vi "Simple VISA Terminal.vi"() -> ()   [LabVIEW 2025]
doc: "Simple string based state machine with internal error handling.\n\n--------------------\n<Author>\n<Company>"
uses:
  <vilib>/Utility/error.llb/Error Cluster From Error Code.vi
  <vilib>/Instr/_visa.llb/VISA Configure Serial Port (Instr).vi
  <vilib>/ErrorRing/Error Ring.xnode
panel:
  in  "Query":bool
  in  "Read":bool
  in  "Write":bool
  in  "VISA resource name":refnum<visa-resource-name>
  in  "Stop":bool
  in  "Start":bool
  in  "Command":string
  out "Error Out":errorcluster
  in  "Error In":errorcluster
  out "Reply":string
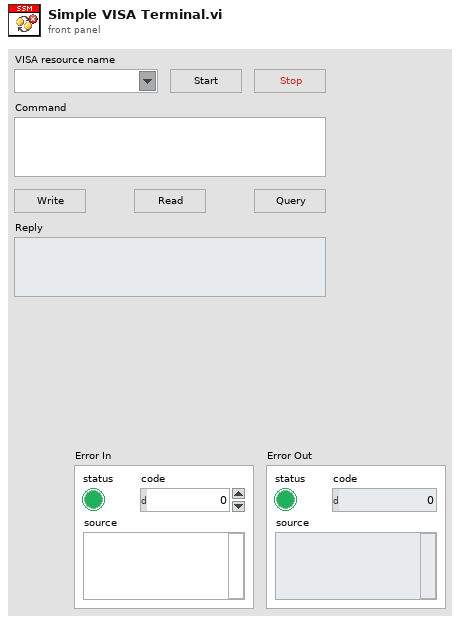
[diagram p1: front panel]
types:
  T1 = cluster{"VISA Reference":refnum<visa-resource-name>, "Reply":string, "Command":string, "Query?":bool}
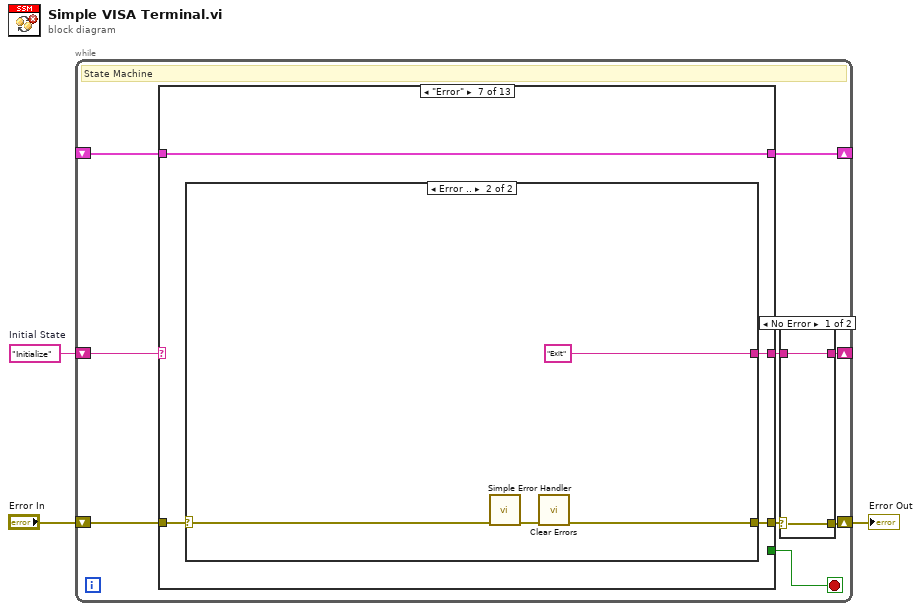
[diagram p0: block diagram]
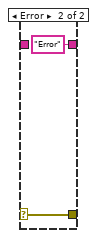
[diagram p2: hidden frame]
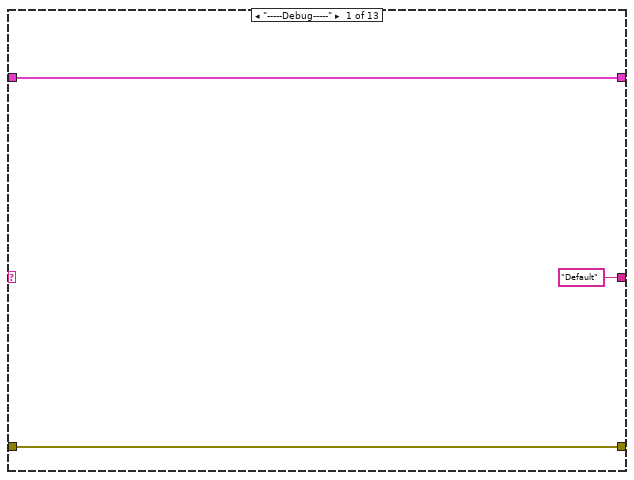
[diagram p3: hidden frame]
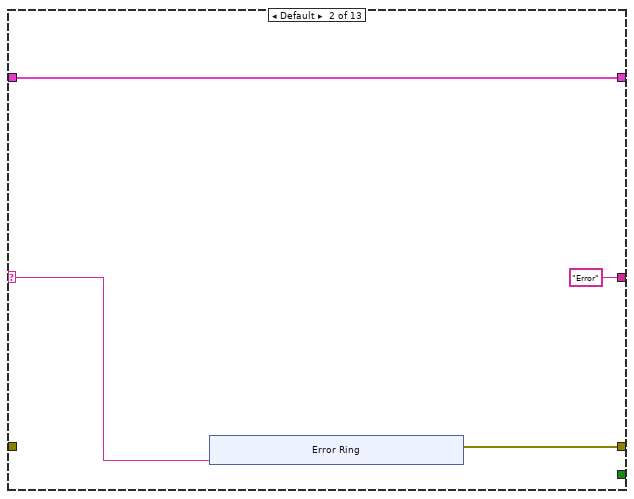
[diagram p4: hidden frame]
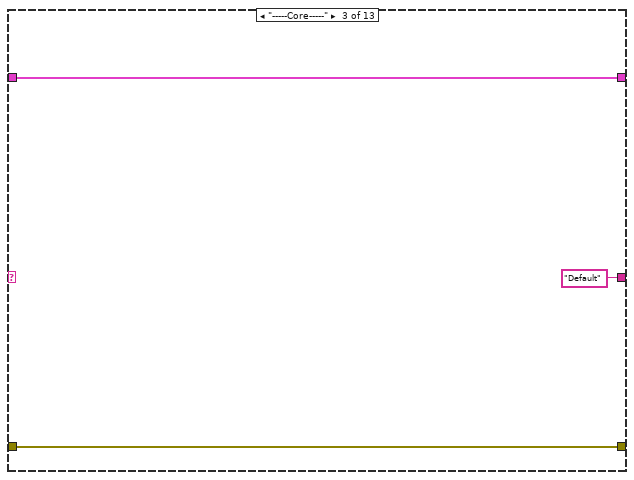
[diagram p5: hidden frame]
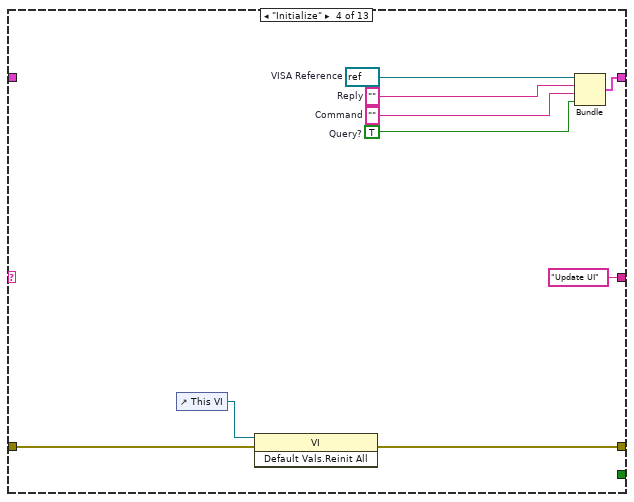
[diagram p6: hidden frame]
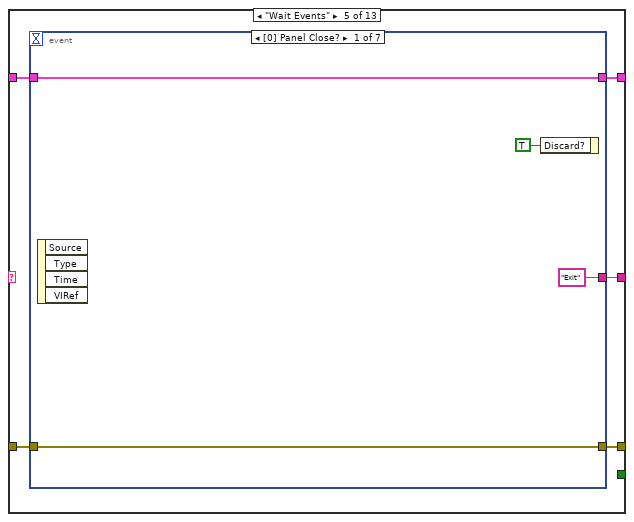
[diagram p7: hidden frame]
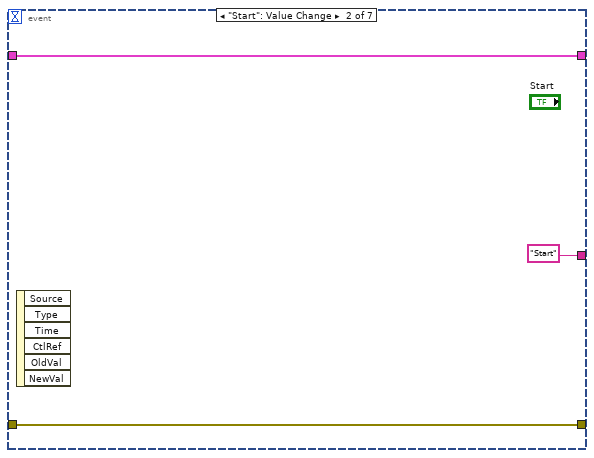
[diagram p8: hidden frame]
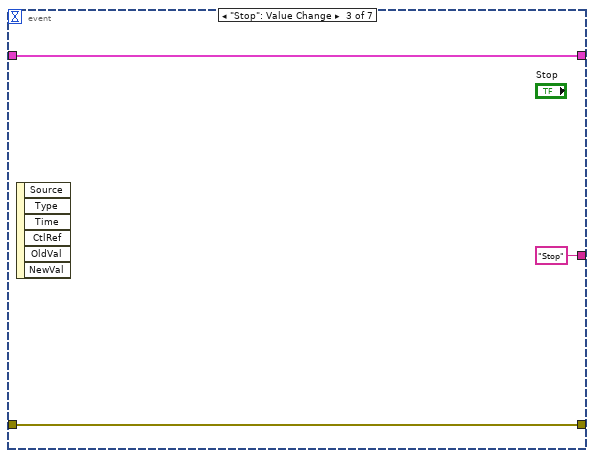
[diagram p9: hidden frame]
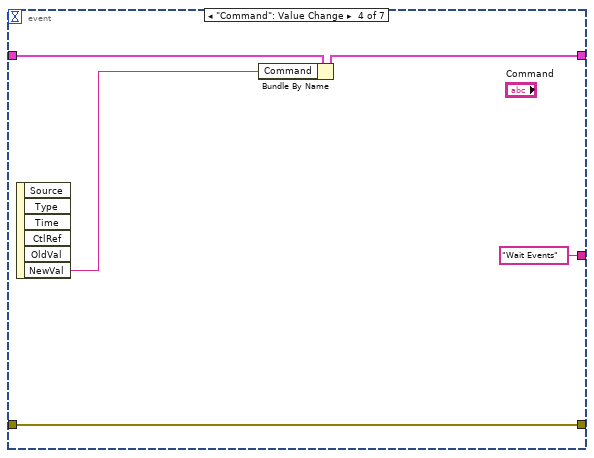
[diagram p10: hidden frame]
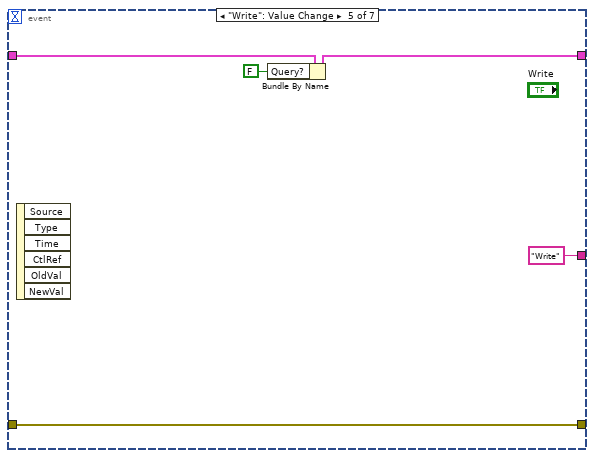
[diagram p11: hidden frame]
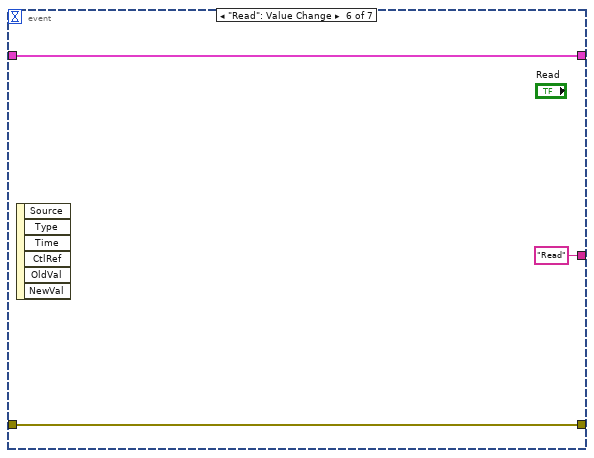
[diagram p12: hidden frame]
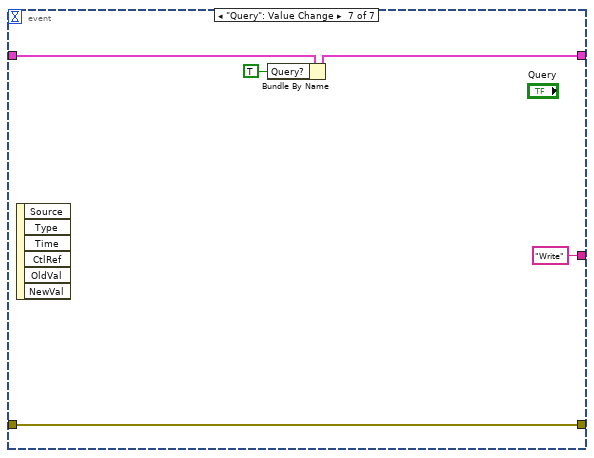
[diagram p13: hidden frame]
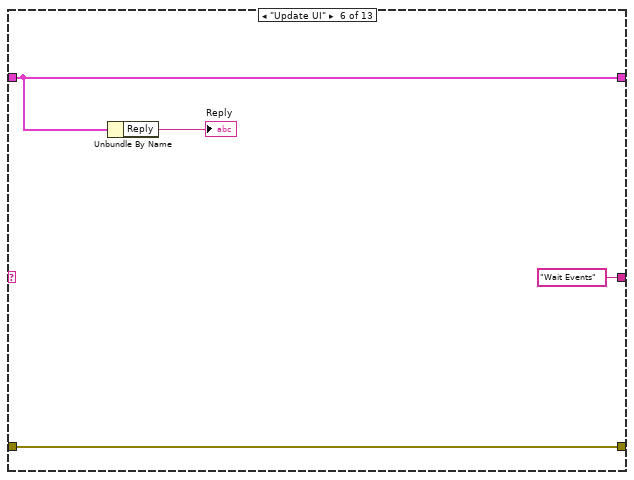
[diagram p14: hidden frame]
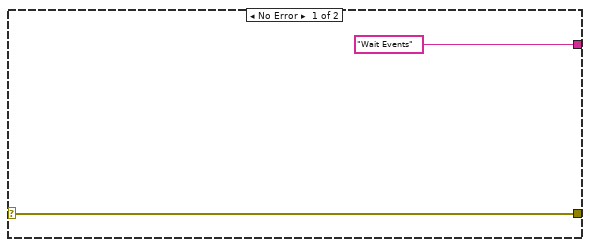
[diagram p15: hidden frame]
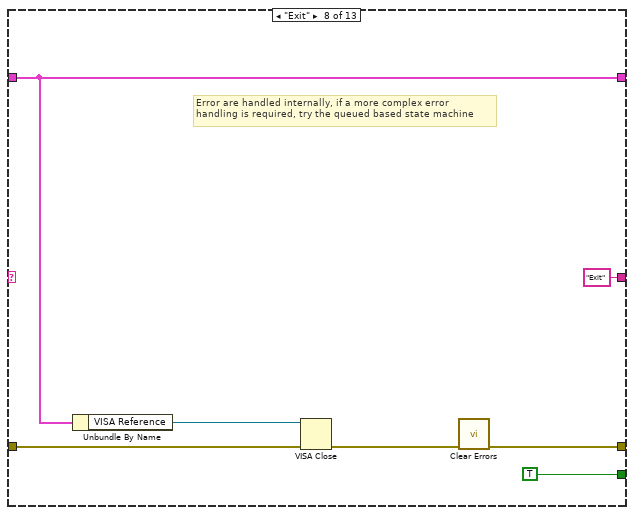
[diagram p16: hidden frame]
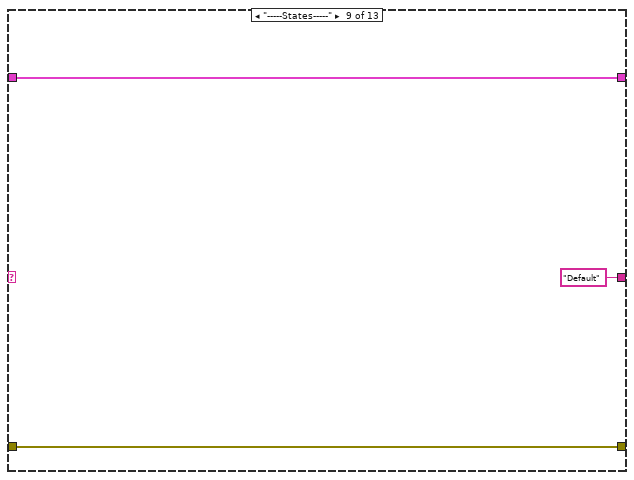
[diagram p17: hidden frame]
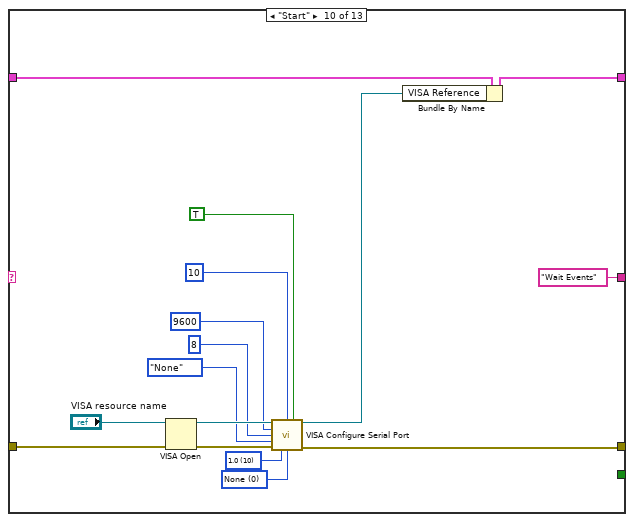
[diagram p18: hidden frame]
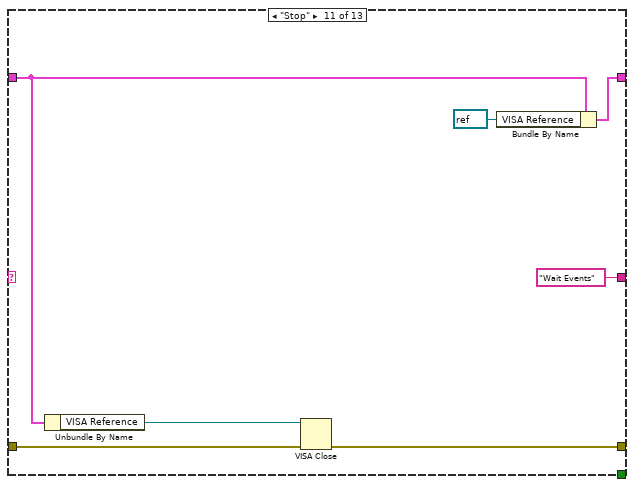
[diagram p19: hidden frame]
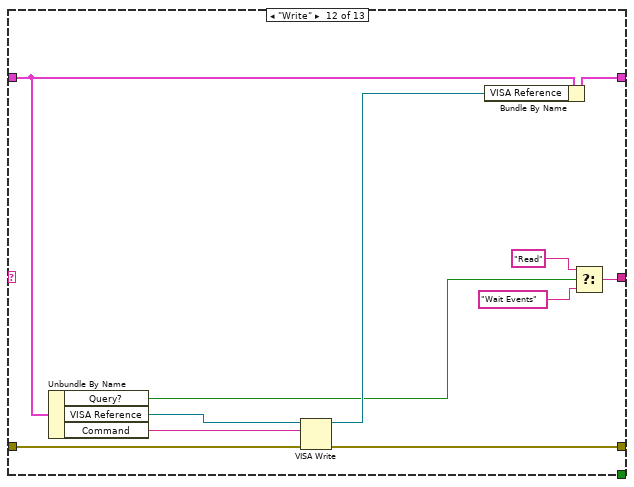
[diagram p20: hidden frame]
diagram:
  w1 = "Initialize"  # Initial State
  n1 = while {
    shift-right: [w4] -> _
    shift-left: w1 -> [w12]
    shift-right: [w10] -> _
    shift-left: _ -> [w11]
    shift-right: [w6] -> w3
    shift-left: "Error In" -> [w8]
    stop <- w9 stop-if-true
    # "State Machine"
    n2 = case shown="\"Error\"" w12 {
      selector: w12 -> [_ w21 _ _ _ _ _ _ _ _ _ _ _]
      tunnel: w8 -> [w19 _ w33 w42 w47 w79 w80 w96 w99 w113 w119 w133 w142]
      tunnel: [w19 w22 w33 w36 w46 w79 w81 w90 w99 w108 w120 w132 w141] -> w7
      tunnel: [_ _ _ _ _ _ _ TRUE _ _ _ _ _] -> w9
      tunnel: ["Default" ("State") "Error" ("Next State") "Default" ("Next State") "Update UI" ("Next State") w45 "Wait Events" ("State") w82 "Exit" ("State") "Default" ("State") "Wait Events" ("State") "Wait Events" ("State") w126 "Update UI" ("State")] -> w5
      tunnel: w11 -> [w18 w23 w32 _ w44 w78 w83 w92 w98 w114 w118 w131 w140]
      tunnel: [w18 w23 w32 w41 w43 w78 w83 w92 w98 w111 w121 w129 w137] -> w10
      frame "-----Debug-----" {
        # "State used for organization purposes."
      }
      frame Default {
        # "Default state used to debug undeclared states."
        n3 = xnode "Error Ring"("parameter 0"=w21) -> ("error out"=w22:errorcluster)
      }
      frame "-----Core-----" {
        # "State used for organization purposes."
      }
      frame "Initialize" {
        w34 = TRUE  # Query?
        w37 = ""  # Command
        w38 = ""  # Reply
        w39 = refnum<visa-resource-name> refnum  # VISA Reference
        # "Initialize the state machine."
        n4 = control-ref of="This VI"() -> (w35:refnum<vi>)
        n5 = invoke class="VI" method="Default Vals.Reinit All"(reference=w35, error in=w42) -> (error out=w36:errorcluster)  [unwired: 1 in, 2 out]
        n6 = Bundle("VISA Reference"=w39, "Reply"=w38, "Command"=w37, "Query?"=w34) -> (w41:T1)  [unwired: 1 in]
      }
      frame "Wait Events" {
        # "Wait for Events"
        n7 = event shown="[0] Panel Close?" {
          selector: _ -> [_ _ _ _ _ _ _]
          dyn-events: _ -> [_ _ _ _ _ _ _]
          timeout: _ -> [_ _ _ _ _ _ _]
          tunnel: w47 -> [w48 w54 w56 w62 w67 w70 w75]
          tunnel: [w48 w54 w56 w62 w67 w70 w75] -> w46
          tunnel: ["Exit" ("State") "Start" ("State") "Stop" ("State") "Wait Events" ("State") "Write" ("State") "Read" ("State") "Write" ("State")] -> w45
          tunnel: w44 -> [w49 w52 w55 w61 w65 w69 w74]
          tunnel: [w49 w52 w55 w59 w64 w69 w72] -> w43
          event Panel Close? {
            # "Stop button value change event."
            n8 = event-data() -> ()  [unwired: 1 in, 4 out]
            n9 = event-data("Discard?"=TRUE) -> ()  [unwired: 1 in, 1 out]
          }
          event "Start": Value Change {
            # "Stop button value change event."
            n10 = event-data() -> ()  [unwired: 1 in, 6 out]
          }
          event "Stop": Value Change {
            # "Ultimate Answer button value change event."
            n11 = event-data() -> ()  [unwired: 1 in, 6 out]
          }
          event "Command": Value Change {
            n12 = event-data() -> ("NewVal"=w58:string)  [unwired: 1 in, 5 out]
            n13 = Bundle By Name(cluster=w61, "Command"=w58) -> (w59:T1)
          }
          event "Write": Value Change {
            # "Ultimate Question button value change event."
            n14 = event-data() -> ()  [unwired: 1 in, 6 out]
            n15 = Bundle By Name(cluster=w65, "Query?"=FALSE) -> (w64:T1)
          }
          event "Read": Value Change {
            n16 = event-data() -> ()  [unwired: 1 in, 6 out]
          }
          event "Query": Value Change {
            n17 = event-data() -> ()  [unwired: 1 in, 6 out]
            n18 = Bundle By Name(cluster=w74, "Query?"=TRUE) -> (w72:T1)
          }
        }
      }
      frame "Update UI" {
        # "Update User Interface"
        n19 = Unbundle By Name(w78) -> ("Reply"=→"Reply":string)
      }
      frame "Error" {
        n20 = case shown="Error .." w80 {
          selector: w80 -> [w85 w89]
          tunnel: [w85 w88] -> w81
          tunnel: ["Wait Events" ("Next State") "Exit" ("Next State")] -> w82
          frame No Error {
          }
          frame Error {
            n21 = call <vilib>:"Simple Error Handler.vi"("error in (no error)"=w89) -> ("error out"=w86:errorcluster)  [unwired: 4 in, 4 out]
            n22 = call <vilib>:"Clear Errors.vi"("error in (no error)"=w86) -> ("error out"=w88:errorcluster)  [unwired: 5 in, 1 out]
          }
        }
      }
      frame "Exit" {
        # "Error are handled internally, if a more complex error\nhandling is required, try the queued based state machine"
        # "Exit the State Machine"
        n23 = Unbundle By Name(w92) -> ("VISA Reference"=w91:refnum<visa-resource-name>)
        n24 = VISA Close(VISA resource name=w91, error in (no error)=w96) -> (error out=w93:errorcluster)
        n25 = call <vilib>:"Clear Errors.vi"("error in (no error)"=w93) -> ("error out"=w90:errorcluster)  [unwired: 5 in, 1 out]
      }
      frame "-----States-----" {
        # "State used for organization purposes."
      }
      frame "Start" {
        w102 = u16 0 items=["None", "XON/XOFF", "RTS/CTS", "XON/XOFF & RTS/CTS", "DTR/DSR", "XON/XOFF & DTR/DSR"] ("flow control (0:none)")
        w103 = u16 10 items=["1.0"=10, "1.5"=15, "2.0"=20] ("stop bits (10: 1 bit)")
        # "Ultimate Answer Event"
        n26 = VISA Open(error in (no error)=w113, VISA resource name="VISA resource name") -> (VISA resource name=w110:refnum<visa-resource-name>, error out=w109:errorcluster)  [unwired: 3 in]
        n27 = call-poly "VISA Configure Serial Port"("VISA resource name"=w110, "termination char\n(0xA = '\\n' = LF)"=u8 10 ("termination char\n(0xA = '\\n' = LF)"), "Enable Termination\nChar (T)"=TRUE ("Enable Termination\nChar (T)"), "baud rate (9600)"=u32 9600, "data bits (8)"=u16 8, "parity (0:none)"=enum16{"None", "Odd", "Even", "Mark", "Space"}."None", "error in (no error)"=w109, "stop bits (10: 1 bit)"=w103, "flow control (0:none)"=w102) -> ("VISA resource name out"=w107:refnum<visa-resource-name>, "error out"=w108:errorcluster)  [unwired: 5 in]
        n28 = Bundle By Name(cluster=w114, "VISA Reference"=w107) -> (w111:T1)
      }
      frame "Stop" {
        # "Ultimate Question Event"
        n29 = Unbundle By Name(w118) -> ("VISA Reference"=w117:refnum<visa-resource-name>)
        n30 = VISA Close(VISA resource name=w117, error in (no error)=w119) -> (error out=w120:errorcluster)
        n31 = Bundle By Name(cluster=w118, "VISA Reference"=refnum<visa-resource-name> refnum) -> (w121:T1)
      }
      frame "Write" {
        n32 = Unbundle By Name(w131) -> ("Query?"=w125:bool, "VISA Reference"=w130:refnum<visa-resource-name>, "Command"=w127:string)
        n33 = VISA Write(VISA resource name=w130, write buffer=w127, error in (no error)=w133) -> (VISA resource name out=w128:refnum<visa-resource-name>, error out=w132:errorcluster)  [unwired: 1 out]
        n34 = Bundle By Name(cluster=w131, "VISA Reference"=w128) -> (w129:T1)
        n35 = Select(t="Read" ("State"), s=w125, f="Wait Events" ("State")) -> (s? t:f=w126:string)
      }
      frame "Read" {
        w138 = u32 1000  # byte count
        n36 = Unbundle By Name(w140) -> ("VISA Reference"=w139:refnum<visa-resource-name>)
        n37 = VISA Read(VISA resource name=w139, byte count=w138, error in (no error)=w142) -> (VISA resource name out=w136:refnum<visa-resource-name>, read buffer=w135:string, error out=w141:errorcluster)  [unwired: 1 out]
        n38 = Bundle By Name(cluster=w140, "VISA Reference"=w136, "Reply"=w135) -> (w137:T1)
      }
    }
    n39 = case shown="No Error" w7 {
      selector: w7 -> [w14 w16]
      tunnel: [w14 w16] -> w6
      tunnel: w5 -> [w13 _]
      tunnel: [w13 "Error" ("State")] -> w4
      frame No Error {
      }
      frame Error {
      }
    }
  }
  "Error Out" <- w3
